vi "get_self_gonghao.vi"(3 "gonghao":string) -> (0 "error 2":errorcluster caption="error out 10", 1 "sp":string[][](array[string]))   [LabVIEW 2017, in "Lib_code.lvlib"]
uses:
  Lib_code.lvlib
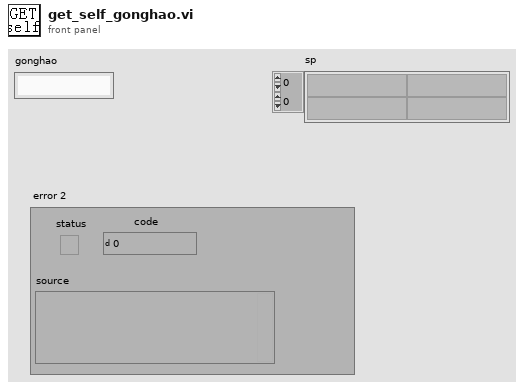
[diagram p1: front panel]
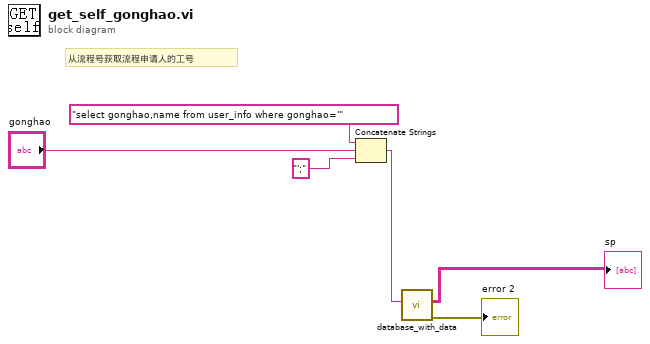
[diagram p0: block diagram]
diagram:
  # "从流程号获取流程申请人的工号"
  n1 = Concatenate Strings("select gonghao,name from user_info where gonghao='" ("Command Text"), "gonghao", "';" ("字符串")) -> (w3:string)
  n2 = call "database_with_data.vi"("input"=w3) -> ("error"=→"error 2":errorcluster, "Data"=→"sp":string[][])  [unwired: 9 in]
